vi "Config External Reference.vi"(0 "VISA Resource Name":refnum<visa-resource-name>, 1 "Standard (0: IS-95A)":T1(ring), 2 "Source (0: Internal)":enum16{"Internal", "External"}(ring), 3 "External Frequency (1.0e+7)":dbl=10000000.0, 5 "error in (no error)":errorcluster {"code" format="%.0x"}) -> (14 "VISA Resource Name Out":refnum<visa-resource-name>, 19 "error out":errorcluster {"code" format="%.0x"})   [LabVIEW 2014, in "Agilent ESG Series.lvlib"]
doc: "This VI configures external reference frequency.\n\nNotes:\n(1) This VI is valid only on instrument E4438C."
uses:
  Agilent ESG Series.lvlib
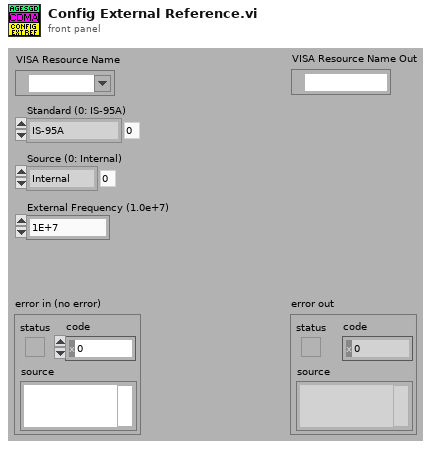
[diagram p1: front panel]
types:
  T1 = enum16{"IS-95A", "CDMA2000", "WCDMA", "Dual Arbitrary"}
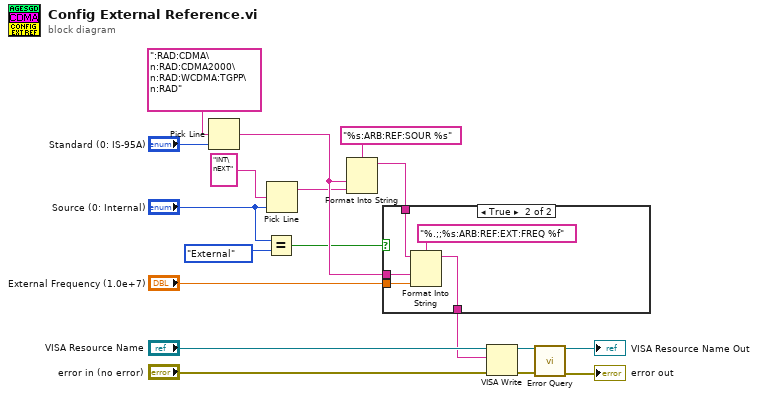
[diagram p0: block diagram]
diagram:
  n1 = Pick Line(multi-line string=":RAD:CDMA\n:RAD:CDMA2000\n:RAD:WCDMA:TGPP\n:RAD", line index="Standard (0: IS-95A)") -> (output string=w10:string)  [unwired: 1 in]
  n2 = Equal?(x="Source (0: Internal)", y=enum16{"Internal", "External"}."External" ("Source (0: Internal)")) -> (x = y?=w5:bool)
  n3 = Pick Line(multi-line string="INT\nEXT", line index="Source (0: Internal)") -> (output string=w1:string)  [unwired: 1 in]
  n4 = Format Into String(format string="%s:ARB:REF:SOUR %s", w10, w1) -> (resulting string=w7:string)  [unwired: 2 in, 1 out]
  n5 = case shown="True" w5 {
    tunnel: w10 -> [_ w23]
    tunnel: "External Frequency (1.0e+7)" -> [_ w22]
    tunnel: w7 -> [w19 w21]
    tunnel: [w19 w20] -> w3
    frame False {
    }
    frame True {
      n6 = Format Into String(format string="%.;;%s:ARB:REF:EXT:FREQ %f", initial string=w21, w23, w22) -> (resulting string=w20:string)  [unwired: 1 in, 1 out]
    }
  }
  n7 = VISA Write(VISA resource name="VISA Resource Name", write buffer=w3, error in (no error)="error in (no error)") -> (VISA resource name out=w14:refnum<visa-resource-name>, error out=w13:errorcluster)  [unwired: 1 out]
  n8 = call "Error Query.vi"("VISA Resource Name"=w14, "error in (no error)"=w13) -> ("VISA Resource Name Out"=→"VISA Resource Name Out":refnum<visa-resource-name>, "error out"=→"error out":errorcluster)  [unwired: 10 in, 2 out]
